vi "refresh_ui.vi"(8 "error in (no error)":errorcluster, 11 "vs_tree_control in":refnum<class "vs_tree_control.lvclass">) -> (0 "error out":errorcluster, 3 "vs_tree_control out":refnum<class "vs_tree_control.lvclass">)   [LabVIEW 2020, in "vs_tree_control.lvclass"]
uses:
  vs_tree_control.lvclass
  vs_tree_control.lvclass/vs_tree_control.ctl
  NationalInstruments.VeriStand.SystemStorageUI
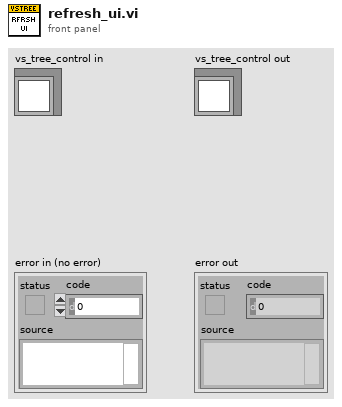
[diagram p1: front panel]
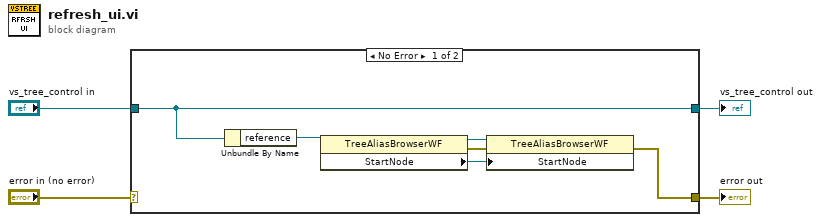
[diagram p0: block diagram]
diagram:
  n1 = case shown="No Error" "error in (no error)" {
    selector: "error in (no error)" -> [_ w12]
    tunnel: [w10 w12] -> w3
    tunnel: [w9 w11] -> w1
    tunnel: "vs_tree_control in" -> [w9 w11]
    frame No Error {
      n2 = Unbundle By Name(w9) -> ("reference"=w8:refnum<k24>)
      n3 = property class="TreeAliasBrowserWF"(reference=w8) -> (reference out=w7:refnum<k24>, error out=w5:errorcluster, "StartNode"=w6:refnum<k24>)  [unwired: 1 in]
      n4 = property class="TreeAliasBrowserWF"(reference=w7, error in=w5, "StartNode"=w6) -> (error out=w10:errorcluster)  [unwired: 1 out]
    }
    frame Error {
    }
  }
  "error out" <- w3
  "vs_tree_control out" <- w1
